vi "Determine Plot Name.vi"(9 "n":i32, 10 "#anchors":i32, 11 "#tags":i32) -> (2 "Plot.Name Array":string[](array[string]))   [LabVIEW 2014]
doc: "This VI determines the name of the plot for plot cosmetics."
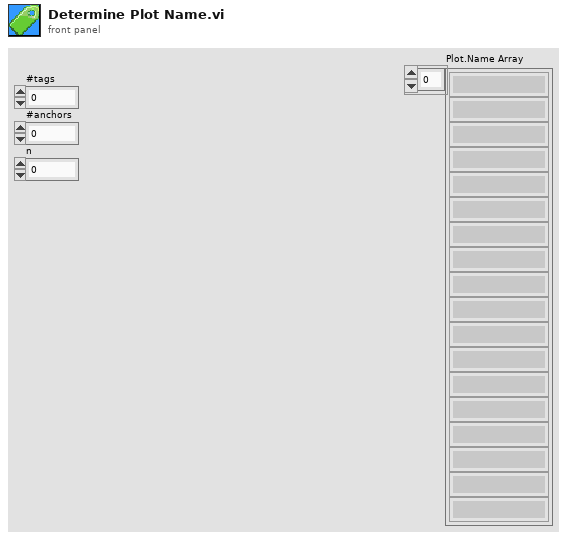
[diagram p1: front panel]
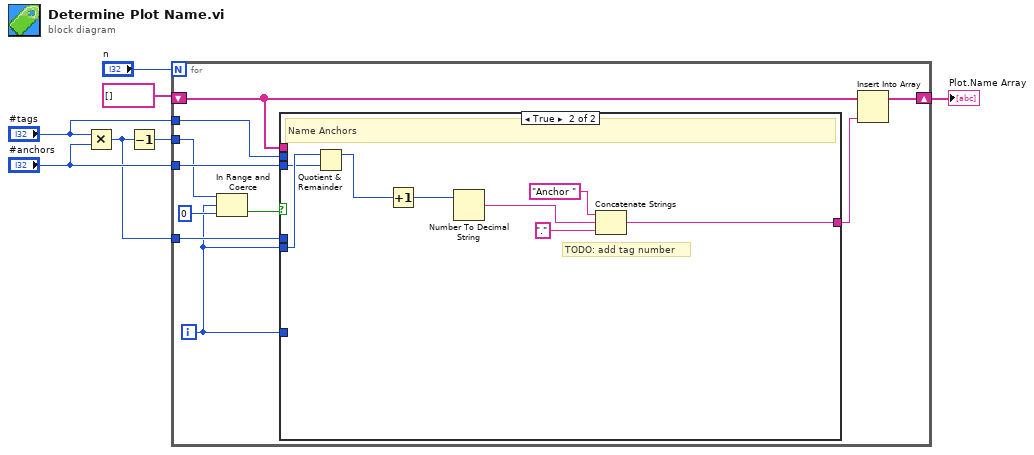
[diagram p0: block diagram]
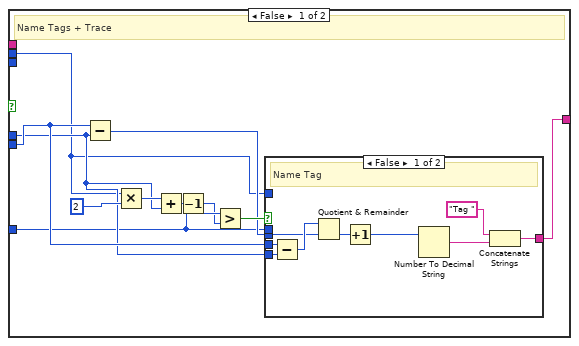
[diagram p2: hidden frame]
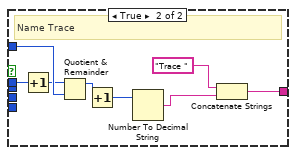
[diagram p3: hidden frame]
diagram:
  n1 = Multiply(x="#tags", y="#anchors") -> (x*y=w1:i32)
  n2 = Decrement(x=w1) -> (x-1=w3:i32)
  n3 = for {
    N: "n" -> [_]
    shift-right: [w17] -> w7
    shift-left: string[] [] ("Plot.Name Array") -> [w9]
    tunnel: w3 -> [w12]
    tunnel: "#anchors" -> [w15]
    tunnel: "#tags" -> [w11]
    tunnel: w1 -> [w10]
    i -> [w8]
    n4 = In Range and Coerce(upper limit=w12, x=w8, lower limit=0) -> (In Range?=w14:bool)  [unwired: 1 out]
    n5 = case shown="True" w14 {
      tunnel: [w21 w52] -> w16
      tunnel: w8 -> [w23 w48]
      tunnel: w15 -> [_ w47]
      tunnel: w11 -> [w20 _]
      tunnel: w10 -> [w22 _]
      tunnel: w9 -> [_ _]
      tunnel: w8 -> [w19 _]
      frame False {
        # "Name Tags + Trace"
        n6 = Subtract(x=w23, y=w22) -> (x-y=w24:i32)
        n7 = Multiply(x=w20, y=2) -> (x*y=w27:i32)
        n8 = Add(x=w27, y=w22) -> (x+y=w26:i32)
        n9 = Decrement(x=w26) -> (x-1=w18:i32)
        n10 = Greater?(x=w19, y=w18) -> (0:w25:bool)
        n11 = case shown="False" w25 {
          tunnel: w24 -> [w33 _]
          tunnel: w23 -> [w32 _]
          tunnel: w22 -> [w31 _]
          tunnel: [w30 w44] -> w21
          tunnel: w20 -> [_ w43]
          tunnel: w19 -> [_ w42]
          frame False {
            # "Name Tag"
            n12 = Subtract(x=w32, y=w31) -> (x-y=w36:i32)
            n13 = Quotient & Remainder(x=w36, y=w33) -> (floor(x/y)=w35:i32)  [unwired: 1 out]
            n14 = Increment(x=w35) -> (x+1=w34:i32)
            n15 = Number To Decimal String(number=w34) -> (decimal integer string=w37:string)  [unwired: 1 in]
            n16 = Concatenate Strings("Tag ", w37) -> (w30:string)
          }
          frame True {
            # "Name Trace"
            n17 = Increment(x=w42) -> (x+1=w39:i32)
            n18 = Quotient & Remainder(x=w39, y=w43) -> (x-y*floor(x/y)=w40:i32)  [unwired: 1 out]
            n19 = Increment(x=w40) -> (x+1=w38:i32)
            n20 = Number To Decimal String(number=w38) -> (decimal integer string=w41:string)  [unwired: 1 in]
            n21 = Concatenate Strings("Trace ", w41) -> (w44:string)
          }
        }
      }
      frame True {
        # "TODO: add tag number"
        # "Name Anchors"
        n22 = Quotient & Remainder(x=w48, y=w47) -> (x-y*floor(x/y)=w49:i32)  [unwired: 1 out]
        n23 = Increment(x=w49) -> (x+1=w46:i32)
        n24 = Number To Decimal String(number=w46) -> (decimal integer string=w51:string)  [unwired: 1 in]
        n25 = Concatenate Strings("Anchor ", w51, ".") -> (w52:string)
      }
    }
    n26 = Insert Into Array(array=w9, new element=w16) -> (w17:string[])  [unwired: 1 in]
  }
  "Plot.Name Array" <- w7
